vi "Close.vi"(8 "error in (no error)":errorcluster, 11 "Instrument in":refnum<class "Instrument.lvclass">) -> (0 "error out":errorcluster, 3 "Instrument out":refnum<class "Instrument.lvclass">)   [LabVIEW 2019, in "Instrument.lvclass"]
uses:
  Instrument.lvclass
  1845f3fb-8aeb-40b3-9131-7f397d222c5c.vi
  1845f3fb-8aeb-40b3-9131-7f397d222c5c.vi/b68bf2f7-dd4a-46cb-9056-d89310eaae54.vi
  RemoteControl/API/Remote Client.vi
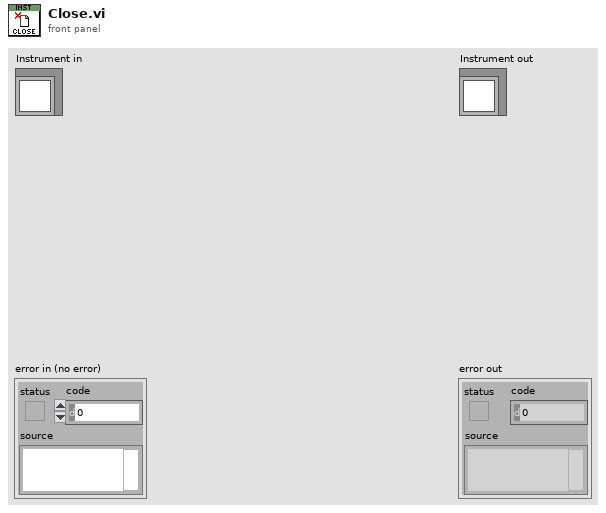
[diagram p1: front panel]
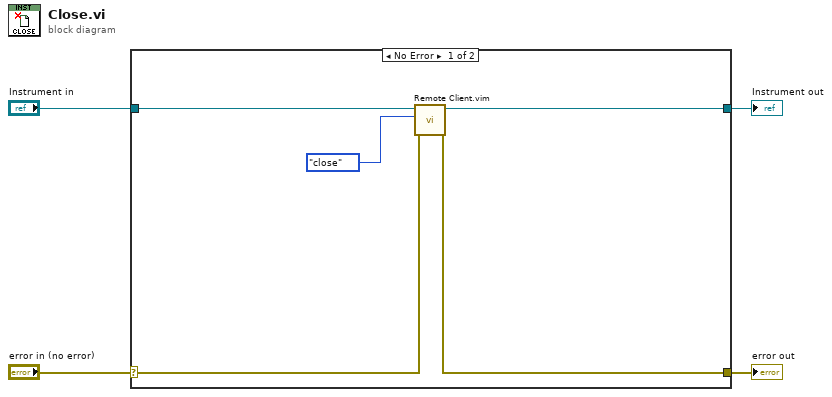
[diagram p0: block diagram]
diagram:
  n1 = case shown="No Error" "error in (no error)" {
    selector: "error in (no error)" -> [w6 w11]
    tunnel: [w8 w11] -> w3
    tunnel: [w9 w10] -> w1
    tunnel: "Instrument in" -> [w7 w10]
    frame No Error {
      n2 = call "Remote Client.vim"("error in (no error)"=w6, "Command"=enum16{"close"}."close", "Instrument in"=w7) -> ("error out"=w8:errorcluster, "Instrument out"=w9:refnum<class "Instrument.lvclass">)  [unwired: 5 in, 2 out]
    }
    frame Error {
    }
  }
  "error out" <- w3
  "Instrument out" <- w1
